vi "MessageAI_State.vi"(8 "Port: 2":u16=20011, 9 "Port:":u16=20011, 10 "SSL Vision Address:":string="127.0.0.1", 11 "IA state":T1={"our_robots"=[], "enemy_robots"=[], "balls"=[], "geometry"={"line_width"=0, "field_length"=0, "field_width"=0, "boundary_width"=0, "referee_width"=0, "goal_width"=0, "goal_depth"=0, "goal_wall_width"=0, "center_circle_radius"=0, "defense_radius"=0, "defense_stretch"=0, "free_kick_from_defense_dist"=0, "penalty_spot_from_field_line_dist"=0, "penalty_line_from_spot_dist"=0}, "IA Judge"={"stage"="", "command"="", "our_goalie_id"=0.0, "enemy_goalie_id"=0.0, "command enum"=enum."Halt", "Time"=enum."Azul"}, "Received Timestamp"=timestamp(0 s since 1904-01-01), "Events"={"Touch"=FALSE, "Ball out"=FALSE, "id touch"=0.0, "Ball out of \nVision"=FALSE, "Ball inside \nGoalie area"=FALSE, "Robot not responding"=FALSE, "Robots responding status"=[1.0, 1.0, 1.0, 1.0, 1.0, 1.0], "Enemy Ball \nPossession"=FALSE, "Pass State"=FALSE, "id end of pass"=0.0, "Kick"=FALSE, "Id ini Possession"=0.0, "Ball Possesion"=FALSE, "Id Possesion"=0.0}}) -> ()   [LabVIEW 2017]
uses:
  Core/AI Input.ctl
  Core/AI Robot.ctl
  Intel/Functions Enum.ctl
  Intel/AttackerStates.ctl
  Path Planning/RRT/PathDests.ctl
  Path Planning/RRT/PathDest.ctl
  Core/AI Ball.ctl
  Core/Field Size.ctl
  Core/AI Judge.ctl
  Intel/Command Enum.ctl
  Util/Events/Events.ctl
panel:
  out "Array 2":u8[](array[numeric])
  out "error out 2":errorcluster
  out "Array":u8[](array[numeric]) format="%02x"
  out "error out":errorcluster
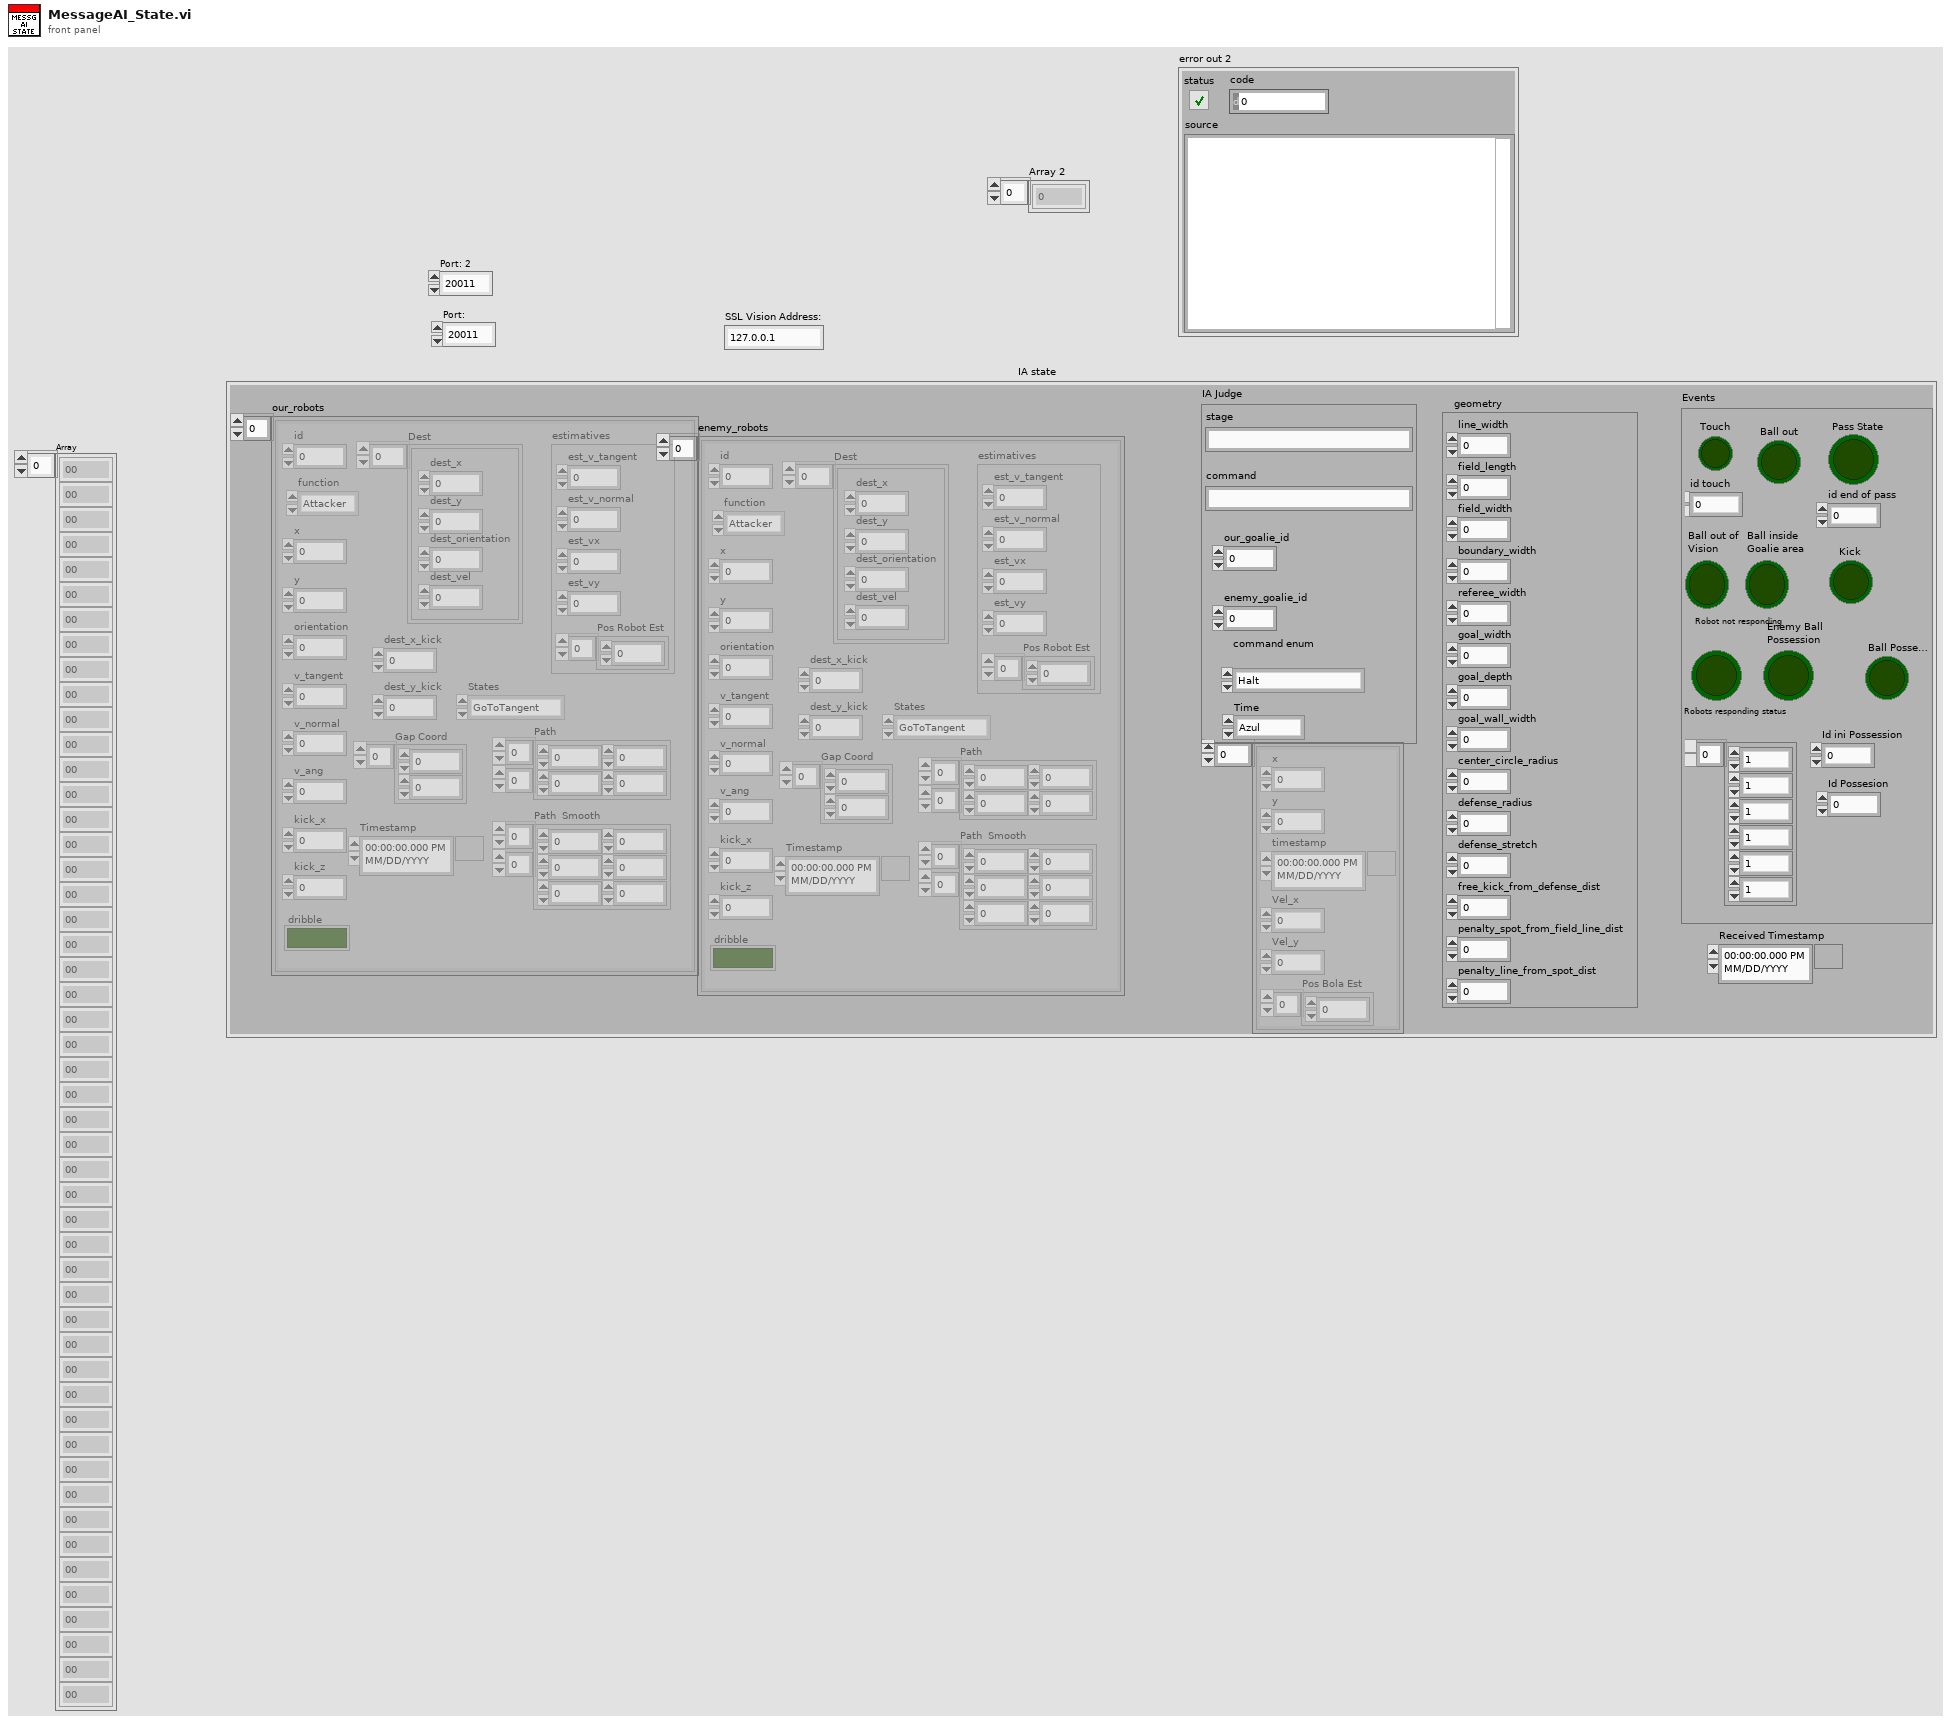
[diagram p1: front panel]
types:
  T1 = typedef "AI Input.ctl" = cluster{"our_robots":T2[], "enemy_robots":T2[], "balls":T7[], "geometry":T8, "IA Judge":T9, "Received Timestamp":timestamp, "Events":T11}
  T2 = typedef "AI Robot.ctl" = cluster{"id":u32, "function":T3, "x":dbl, "y":dbl, "orientation":dbl, "v_tangent":dbl, "v_normal":dbl, "v_ang":dbl, "kick_x":dbl, "kick_z":dbl, "dribble":bool, "Timestamp":timestamp, "estimatives":cluster{"est_v_tangent":dbl, "est_v_normal":dbl, "est_vx":dbl, "est_vy":dbl, "Pos Robot Est":dbl[]}, "dest_x_kick":dbl, "dest_y_kick":dbl, "Gap Coord":dbl[], "States":T4, "Path ":dbl[][], "Path  Smooth":dbl[][], "Dest":T5}
  T3 = typedef "Functions Enum.ctl" = enum16{"Attacker", "Goalie", "Defender", "Striker", "Goto 0", "Dummy", "Kicker", "ZigZag"}
  T4 = typedef "AttackerStates.ctl" = enum16{"Pass", "GoToTangent", "BallGetting", "GoToKick", ""}
  T5 = typedef "PathDests.ctl" = T6[]
  T6 = typedef "PathDest.ctl" = cluster{"dest_x":dbl, "dest_y":dbl, "dest_orientation":dbl, "dest_vel":dbl}
  T7 = typedef "AI Ball.ctl" = cluster{"x":dbl, "y":dbl, "timestamp":timestamp, "Vel_x":dbl, "Vel_y":dbl, "Pos Bola Est":dbl[]}
  T8 = typedef "Field Size.ctl" = cluster{"line_width":u32, "field_length":u32, "field_width":u32, "boundary_width":u32, "referee_width":u32, "goal_width":u32, "goal_depth":u32, "goal_wall_width":u32, "center_circle_radius":u32, "defense_radius":u32, "defense_stretch":u32, "free_kick_from_defense_dist":u32, "penalty_spot_from_field_line_dist":u32, "penalty_line_from_spot_dist":u32}
  T9 = typedef "AI Judge.ctl" = cluster{"stage":string, "command":string, "our_goalie_id":dbl, "enemy_goalie_id":dbl, "command enum":T10, "Time":enum16{"Azul", "Amarelo"}}
  T10 = typedef "Command Enum.ctl" = enum16{"Halt", "Stop", "Force Start", "PKA Normal Start", "Prepare Kickoff Ally", "PKE Normal Start", "Prepare Kickoff Enemy", "Prepare Penalty Ally", "PPA Normal Start", "Prepare Penalty Enemy", "PPE Normal Start", "Direct Free Enemy", "Direct Free Ally", "Indirect Free Enemy", "Indirect Free Ally", "Timeout Enemy", "Timeout Ally", "Goal Enemy", "Goal Ally", "Ball Placement Enemy", "Ball Placement Ally", "Normal Half Time", "Extra Time Break", "Extra Half Time", "None", "Post Game"}
  T11 = typedef "Events.ctl" = cluster{"Touch":bool, "Ball out":bool, "id touch":dbl, "Ball out of \nVision":bool, "Ball inside \nGoalie area":bool, "Robot not responding":bool, "Robots responding status":dbl[], "Enemy Ball \nPossession":bool, "Pass State":bool, "id end of pass":dbl, "Kick":bool, "Id ini Possession":dbl, "Ball Possesion":bool, "Id Possesion":dbl}
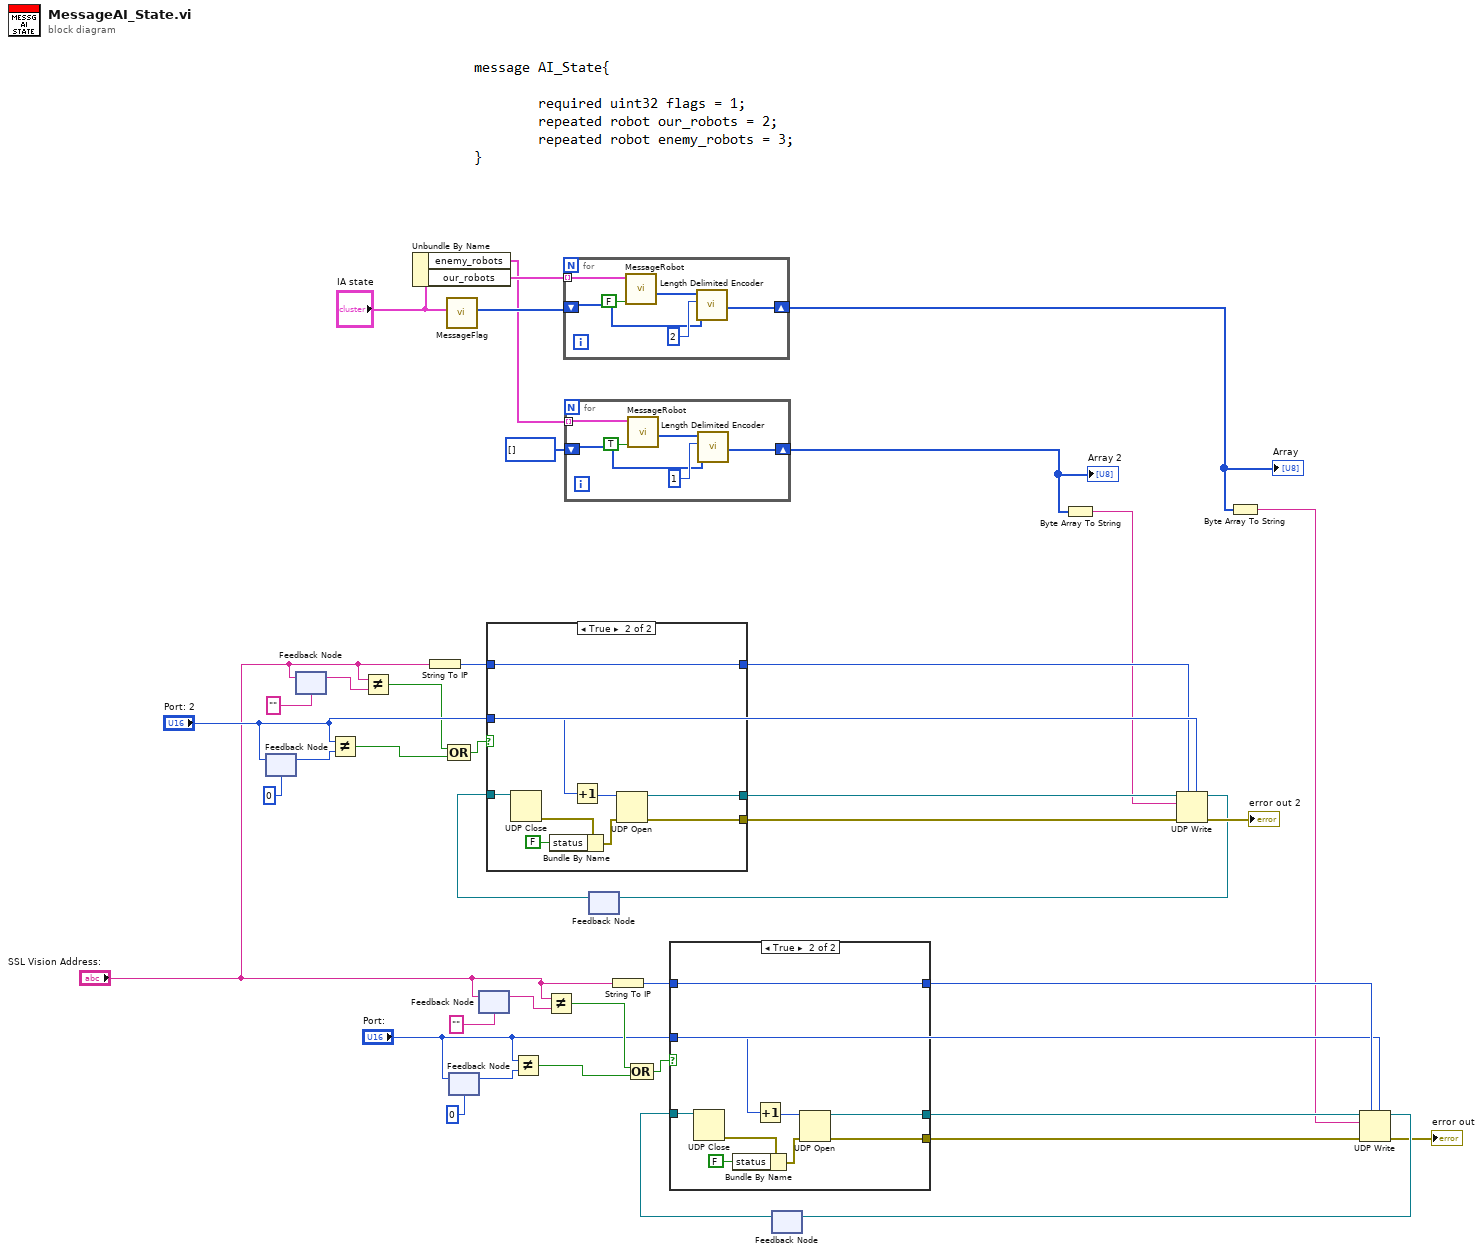
[diagram p0: block diagram]
diagram:
  n1 = feedback #1(u16 0 ("Port:")) -> (w18:u16)
  n2 = feedback-in #1("Port: 2") -> ()
  n3 = feedback #2("" ("SSL Vision Address:")) -> (w16:string)
  n4 = feedback-in #2("SSL Vision Address:") -> ()
  n5 = Not Equal?(x="Port: 2", y=w18) -> (x != y?=w14:bool)
  n6 = Not Equal?(x="SSL Vision Address:", y=w16) -> (x != y?=w15:bool)
  n7 = Unbundle By Name("IA state") -> ("enemy_robots"=w21:T2[], "our_robots"=w22:T2[])
  n8 = String To IP(1:"SSL Vision Address:") -> (0:w6:u32)
  n9 = call "MessageFlag.vi"("input cluster"="IA state") -> ("Array"=w24:u8[])  [unwired: 10 in]
  n10 = Compound Arithmetic op=OR(w15, w14) -> (w13:bool)
  n11 = feedback #3(u16 0 ("Port:")) -> (w27:u16)
  n12 = feedback-in #3("Port:") -> ()
  n13 = feedback #4("" ("SSL Vision Address:")) -> (w29:string)
  n14 = feedback-in #4("SSL Vision Address:") -> ()
  n15 = Not Equal?(x="Port:", y=w27) -> (x != y?=w31:bool)
  n16 = Not Equal?(x="SSL Vision Address:", y=w29) -> (x != y?=w30:bool)
  n17 = for {
    shift-right: [w46] -> w20
    shift-left: w24 -> [w44]
    tunnel: w22 -> [w43] mode=indexing
    n18 = call "MessageRobot.vi"("Enemy Robots?"=FALSE, "Robot"=w43) -> ("Array"=w42:u8[])  [unwired: 9 in]
    n19 = call "Length Delimited Encoder.vi"("Array In"=w44, "Key"=u32 2, "Array In 2"=w42) -> ("Array"=w46:u8[])  [unwired: 8 in]
  }
  "Array" <- w20
  n20 = for {
    shift-right: [w52] -> w4
    shift-left: u8[] [] ("Array") -> [w50]
    tunnel: w21 -> [w49] mode=indexing
    n21 = call "MessageRobot.vi"("Enemy Robots?"=TRUE, "Robot"=w49) -> ("Array"=w48:u8[])  [unwired: 9 in]
    n22 = call "Length Delimited Encoder.vi"("Array In"=w50, "Key"=u32 1, "Array In 2"=w48) -> ("Array"=w52:u8[])  [unwired: 8 in]
  }
  "Array 2" <- w4
  n23 = feedback #5() -> (w11:refnum<k16>)  [unwired: 1 in]
  n24 = case shown="True" w13 {
    tunnel: [_ w63] -> w19
    tunnel: [w54 w61] -> w10
    tunnel: "Port: 2" -> [_ w60]
    tunnel: w6 -> [w53 w58]
    tunnel: w11 -> [w54 w59]
    tunnel: [w53 w58] -> w5
    frame False {
    }
    frame True {
      n25 = UDP Close(connection ID=w59) -> (error out=w57:errorcluster)  [unwired: 1 in, 1 out]
      n26 = Bundle By Name(cluster=w57, "status"=FALSE) -> (w56:errorcluster)
      n27 = Increment(x=w60) -> (x+1=w62:u16)
      n28 = UDP Open(8:w56, 11:w62) -> (port=w61:refnum<k16>, 0:w63:errorcluster)  [unwired: 3 in, 1 out]
    }
  }
  n29 = String To IP(1:"SSL Vision Address:") -> (0:w39:u32)
  n30 = Compound Arithmetic op=OR(w30, w31) -> (w32:bool)
  n31 = feedback #6() -> (w34:refnum<k16>)  [unwired: 1 in]
  n32 = case shown="True" w32 {
    tunnel: [_ w74] -> w26
    tunnel: [w65 w72] -> w35
    tunnel: "Port:" -> [_ w71]
    tunnel: w39 -> [w64 w69]
    tunnel: w34 -> [w65 w70]
    tunnel: [w64 w69] -> w40
    frame False {
    }
    frame True {
      n33 = UDP Close(connection ID=w70) -> (error out=w68:errorcluster)  [unwired: 1 in, 1 out]
      n34 = Bundle By Name(cluster=w68, "status"=FALSE) -> (w67:errorcluster)
      n35 = Increment(x=w71) -> (x+1=w73:u16)
      n36 = UDP Open(8:w67, 11:w73) -> (port=w72:refnum<k16>, 0:w74:errorcluster)  [unwired: 3 in, 1 out]
    }
  }
  n37 = Byte Array To String(unsigned byte array=w4) -> (string=w3:string)
  n38 = UDP Write(address=w5, port or service name="Port: 2", connection ID=w10, data in=w3, 8:w19) -> (error out=→"error out 2":errorcluster, 3:w9:refnum<k16>)  [unwired: 1 in]
  n39 = feedback-in #5(w9) -> ()
  n40 = Byte Array To String(unsigned byte array=w20) -> (string=w25:string)
  n41 = UDP Write(address=w40, port or service name="Port:", connection ID=w35, data in=w25, 8:w26) -> (error out=→"error out":errorcluster, 3:w36:refnum<k16>)  [unwired: 1 in]
  n42 = feedback-in #6(w36) -> ()
